vi "Cache Failed Data Point.vi"(0 "Reset?":bool, 3 "Current Cache":T1[](array[typedef]), 4 "New Cache":T1, 5 "Channels Size":i32, 6 "Channel Index":i32, 7 "error in (no error)":errorcluster) -> (20 "Cache out":T1[](array[typedef]), 27 "error out":errorcluster)   [LabVIEW 2026, in "Processing_Engine.lvlib"]
doc: "Overwrite current failed data point with new failed data point into cache."
uses:
  Processing_Engine.lvlib
  controls/Messaging Payloads/Processed Calibration Point.ctl
  controls/UI/Direction.ctl
  Test Status.ctl
  Settings/Settings.lvlib
  Analysis/Analysis.lvlib
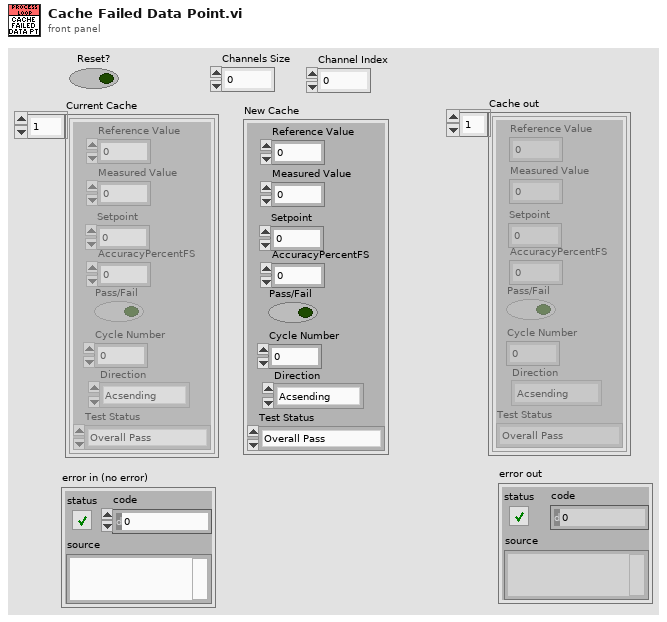
[diagram p1: front panel]
types:
  T1 = typedef "Processed Calibration Point.ctl" = cluster{"Reference Value":dbl, "Measured Value":dbl, "AccuracyPercentFS":dbl, "Pass/Fail":bool, "Setpoint":dbl, "Cycle Number":i32, "Direction":T2, "Test Status":T3}
  T2 = typedef "Settings.lvlib/Direction.ctl" = enum16{"Acsending", "Descending"}
  T3 = typedef "Analysis.lvlib/Test Status.ctl" = enum16{"Overall Pass", "Overall Fail", "Test Running"}
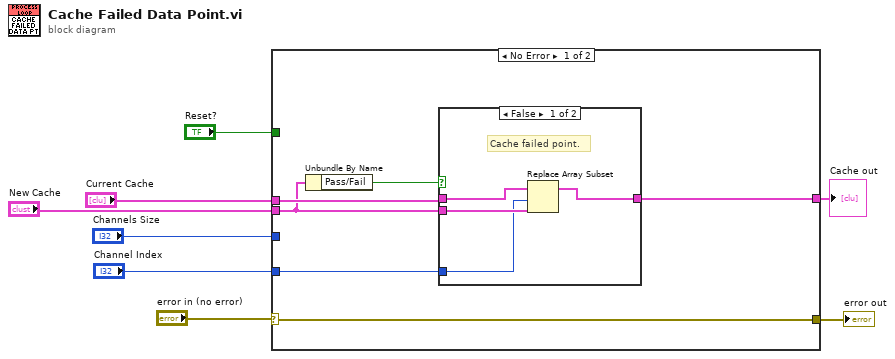
[diagram p0: block diagram]
diagram:
  n1 = case shown="No Error" "error in (no error)" {
    selector: "error in (no error)" -> [w12 w21]
    tunnel: "Current Cache" -> [w14 w20]
    tunnel: [w13 w20] -> w2
    tunnel: "New Cache" -> [w9 _]
    tunnel: [w12 w21] -> w5
    tunnel: "Reset?" -> [_ _]
    tunnel: "Channels Size" -> [_ _]
    tunnel: "Channel Index" -> [w11 _]
    frame No Error {
      n2 = Unbundle By Name(w9) -> ("Pass/Fail"=w10:bool)
      n3 = case shown="False" w10 {
        tunnel: w9 -> [w18 _]
        tunnel: [w16 w19] -> w13
        tunnel: w14 -> [w17 w19]
        tunnel: w11 -> [w15 _]
        frame False {
          # "Cache failed point."
          n4 = Replace Array Subset(array=w17, new element=w18, index=w15) -> (w16:T1[])
        }
        frame True {
          # "Maintain failed cache."
        }
      }
    }
    frame Error {
    }
  }
  "error out" <- w5
  "Cache out" <- w2
